vi "Table, Set Cell Text Plain.vi"(6 "error in":errorcluster, 7 "col (0)":i32, 8 "row (0)":i32, 9 "Tbl Refnum":refnum<vi>) -> (0 "error out":errorcluster, 1 "col+1":i32=-1, 2 "row+1":i32=-1, 3 "Tbl Refnum out":refnum<vi>)   [LabVIEW 2010]
doc: "This function sets the active table cell font attribute to bold."
uses:
  <vilib>/Utility/miscctls.llb/LVRowAndColumnTypeDef.ctl
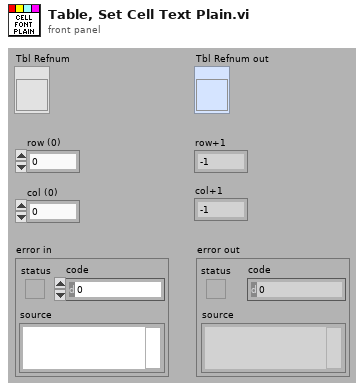
[diagram p1: front panel]
types:
  T1 = typedef "LVRowAndColumnTypeDef.ctl" = cluster{"Row":i32, "Column":i32}
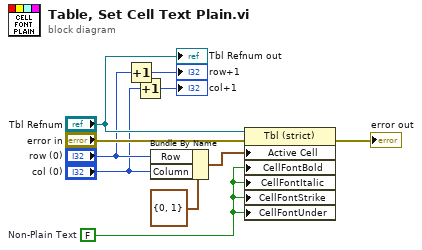
[diagram p0: block diagram]
diagram:
  w1 = FALSE  # Non-Plain Text
  n1 = Increment(x="row (0)") -> (x+1=→"row+1":i32)
  n2 = Increment(x="col (0)") -> (x+1=→"col+1":i32)
  n3 = Bundle By Name(cluster=T1 {"Row"=0, "Column"=1} ("Selection Start 2"), "Row"="row (0)", "Column"="col (0)") -> (w7:T1)
  n4 = property class="Tbl (strict)"(reference="Tbl Refnum", error in="error in", "Active Cell"=w7, "CellFontBold"=w1, "CellFontItalic"=w1, "CellFontStrike"=w1, "CellFontUnder"=w1) -> (error out=→"error out":errorcluster)  [unwired: 1 out]
  "Tbl Refnum out" <- "Tbl Refnum"
